vi "Reset Output Protection.vi"(8 "error in (no error)":errorcluster, 11 "VISA resource name":refnum<visa-resource-name>) -> (0 "error out":errorcluster, 3 "VISA resource name out":refnum<visa-resource-name>)   [LabVIEW 2020, in "RIGOL DP800 Series.lvlib"]
doc: "Resets the status of over voltage protection (OVP) and over current protection (OCP)."
uses:
  <instrlib>/RIGOL DP800 Series/RIGOL DP800 Series.lvlib
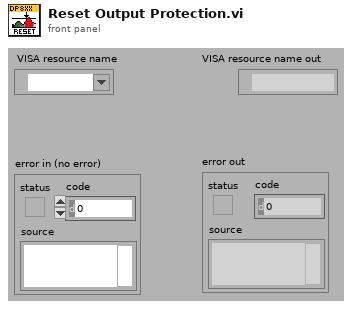
[diagram p1: front panel]
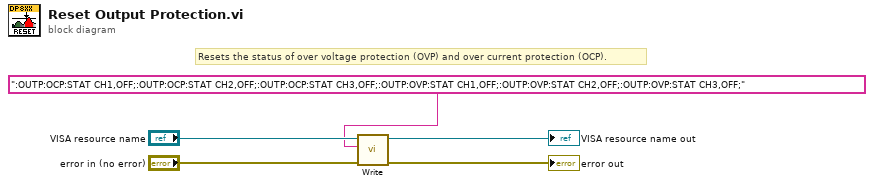
[diagram p0: block diagram]
diagram:
  # "Resets the status of over voltage protection (OVP) and over current protection (OCP)."
  n1 = call <instrlib>:"Write.vi"("error in (no error)"="error in (no error)", "Write Buffer (\"\")"=":OUTP:OCP:STAT CH1,OFF;:OUTP:OCP:STAT CH2,OFF;:OUTP:OCP:STAT CH3,OFF;:OUTP:OVP:STAT CH1,OFF;:OUTP:OVP:STAT CH2,OFF;:OUTP:OVP:STAT CH3,OFF;", "VISA resource name"="VISA resource name") -> ("error out"=→"error out":errorcluster, "VISA resource name out"=→"VISA resource name out":refnum<visa-resource-name>)  [unwired: 7 in]
